vi "Julian_project3.vi"() -> ()   [LabVIEW 2020]
uses:
  Control 2.ctl
panel:
  out "Numeric 3":dbl
  out "Total 2":dbl
  out "Time 2":dbl
  in  "Cluster 2":T1
  out "Numeric":dbl
  out "Numeric 2":dbl
  # "time"
  # "Lap Time"
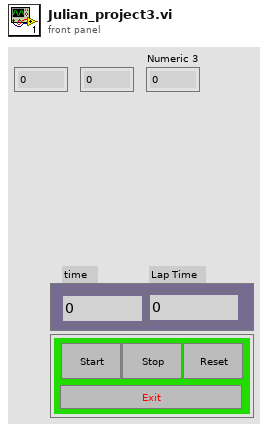
[diagram p1: front panel]
types:
  T1 = cluster{"Stop":bool, "Reset":bool, "Exit":bool, "Start":bool}
  T2 = typedef "Control 2.ctl" = enum16{"idle", "Run", "wait", "reset"}
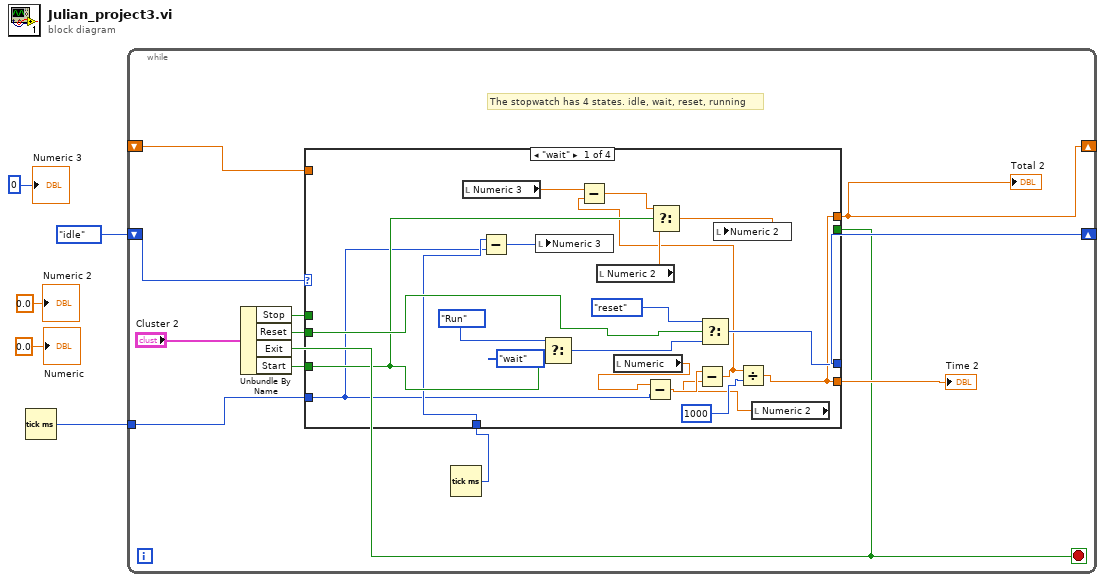
[diagram p0: block diagram]
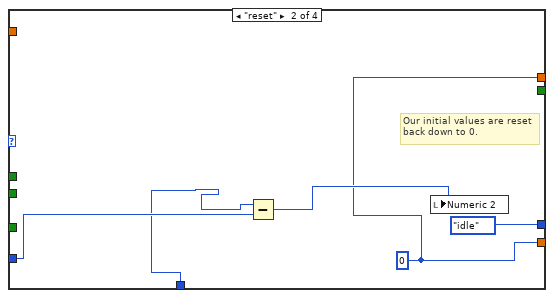
[diagram p2: hidden frame]
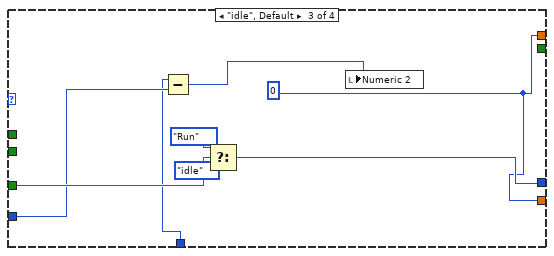
[diagram p3: hidden frame]
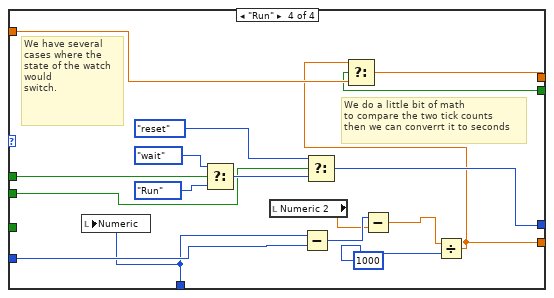
[diagram p4: hidden frame]
diagram:
  n1 = Tick Count (ms)() -> (millisecond timer value=w4:u32)
  n2 = while {
    tunnel: w4 -> [w11]
    shift-right: [w13] -> _
    shift-left: Control_2."idle" -> [w17]
    shift-right: [w9] -> _
    shift-left: _ -> [w7]
    stop <- w6 stop-if-true
    # "The stopwatch has 4 states. idle, wait, reset, running"
    n3 = Unbundle By Name("Cluster 2") -> ("Stop"=w16:bool, "Reset"=w15:bool, "Exit"=w6:bool, "Start"=w14:bool)
    n4 = Tick Count (ms)() -> (millisecond timer value=w12:u32)
    n5 = case shown="\"wait\"" w17 {
      tunnel: w16 -> [_ _ _ w62]
      tunnel: w15 -> [w34 _ _ w52]
      tunnel: [w28 Control_2."idle" w48 w63] -> w13
      tunnel: w14 -> [w25 _ w47 _]
      tunnel: [w27 w38 w43 w54] -> w9
      tunnel: w11 -> [w21 w41 w45 w61]
      tunnel: [w27 w38 w43 w55] -> w8
      tunnel: w12 -> [w22 w40 w44 w57]
      tunnel: w7 -> [_ _ _ w56]
      tunnel: w6 -> [_ _ _ w53]
      frame "wait" {
        n6 = local read "Numeric 3"() -> (w20:dbl)
        n7 = Subtract(x=w22, y=w21) -> (x-y=w26:u32)
        n8 = local write "Numeric 3"(w26) -> ()
        n9 = Select(t=Control_2."Run", s=w25, f=Control_2."wait") -> (s? t:f=w33:T2)
        n10 = local read "Numeric 2"() -> (w24:dbl)
        n11 = local read "Numeric"() -> (w32:dbl)
        n12 = Subtract(x=w32, y=w21) -> (x-y=w30:dbl)
        n13 = Select(t=Control_2."reset", s=w34, f=w33) -> (s? t:f=w28:T2)
        n14 = local read "Numeric 2"() -> (w29:dbl)
        n15 = Subtract(x=w30, y=w29) -> (x-y=w18:dbl)
        n16 = Subtract(x=w20, y=w18) -> (x-y=w19:dbl)
        n17 = Select(t=w19, s=w25, f=w24) -> (s? t:f=w23:dbl)
        n18 = local write "Numeric 2"(w23) -> ()
        n19 = Divide(x=w18, y=1000) -> (x/y=w27:dbl)
      }
      frame "reset" {
        w38 = 0
        # "Our initial values are reset\nback down to 0."
        n20 = Subtract(x=w40, y=w41) -> (x-y=w39:u32)
        n21 = local write "Numeric 2"(w39) -> ()
      }
      frame "idle", Default {
        w43 = u32 0 ("x")
        n22 = Subtract(x=w44, y=w45) -> (x-y=w46:u32)
        n23 = Select(t=Control_2."Run", s=w47, f=Control_2."idle") -> (s? t:f=w48:T2)
        n24 = local write "Numeric 2"(w46) -> ()
      }
      frame "Run" {
        # "We have several\ncases where the \nstate of the watch would \nswitch."
        # "We do a little bit of math \nto compare the two tick counts\nthen we can converrt it to seconds"
        n25 = local write "Numeric"(w57) -> ()
        n26 = Select(t=Control_2."wait", s=w62, f=Control_2."Run") -> (s? t:f=w65:T2)
        n27 = local read "Numeric 2"() -> (w58:dbl)
        n28 = Subtract(x=w57, y=w61) -> (x-y=w59:u32)
        n29 = Select(t=Control_2."reset", s=w52, f=w65) -> (s? t:f=w63:T2)
        n30 = Subtract(x=w59, y=w58) -> (x-y=w51:dbl)
        n31 = Divide(x=w51, y=1000) -> (x/y=w55:dbl)
        n32 = Select(t=w55, s=w53, f=w56) -> (s? t:f=w54:dbl)
      }
    }
    "Total 2" <- w9
    "Time 2" <- w8
  }
  "Numeric 2" <- 0.0 ("Numeric 2")
  "Numeric" <- 0.0 ("Numeric")
  "Numeric 3" <- 0
